vi "rsscope_core_global.vi"() -> ()   [LabVIEW 2014] (continued)
"Class Only"=FALSE, "Identifier"="RSSCOPE_ATTR_MASK_CONVERT_TO_USER", "Descriptive Name"="Mask Test Convert To User", "Data Type"=2, "Command"="MTES:CEM", "Access"=1, "Range Table"="", "Read Callback"="", "Write Callback"="", "Supported Models"="", "Instrument Options"="", "Flags"=0, "Help"="Converts the test and mask definitions of the current mask test to a new mask test of type User.\n\nAvailable Repeated Capabilities:\nNone\n\nRemote-control command(s):\nMTESt:CEMask"}, {"Level"=3, "Class Only"=FALSE, "Identifier"="RSSCOPE_ATTR_MASK_TEST_ENABLE", "Descriptive Name"="Mask Test Enable", "Data Type"=3, "Command"="MTES", "Access"=2, "Range Table"="", "Read Callback"="rsscope_formatMaskNameBoolean_ReadCallback.vi", "Write Callback"="rsscope_formatMaskNameBoolean_WriteCallback.vi", "Supported Models"="", "Instrument Options"="", "Flags"=0, "Help"="This attribute activates and deactivates the mask test.\n\nAvailable Repeated Capabilities:\nNone\n\nRemote-control command(s):\nMTESt[:STATe]"}, {"Level"=3, "Class Only"=FALSE, "Identifier"="RSSCOPE_ATTR_MASK_TEST_CLEAR_ALL", "Descriptive Name"="Mask Test Clear All", "Data Type"=4, "Command"="MTES:RST", "Access"=1, "Range Table"="", "Read Callback"="", "Write Callback"="", "Supported Models"="", "Instrument Options"="", "Flags"=0, "Help"="Clears all totals and results in all &apos;Mask Test&apos; result boxes.\n\nAvailable Repeated Capabilities:\nNone\n\nRemote-control command(s):\nMTESt:RST"}, {"Level"=3, "Class Only"=FALSE, "Identifier"="RSSCOPE_ATTR_MASK_TEST_DEFINITION_TYPE", "Descriptive Name"="Mask Test Definition Type", "Data Type"=0, "Command"="MTES:CTYP", "Access"=2, "Range Table"="RsScope_rngMaskTestDefinitionType", "Read Callback"="rsscope_formatMaskNameInt32_ReadCallback.vi", "Write Callback"="rsscope_formatMaskNameInt32_WriteCallback.vi", "Supported Models"="", "Instrument Options"="", "Flags"=0, "Help"="This control selects the method of mask definition.\n\nAvailable Repeated Capabilities:\nNone\n\nRemote-control command(s):\nMTESt:CTYPe"}, {"Level"=3, "Class Only"=FALSE, "Identifier"="RSSCOPE_ATTR_MASK_TEST_SOURCE", "Descriptive Name"="Mask Test Source", "Data Type"=0, "Command"="MTES:SOUR", "Access"=2, "Range Table"="rsscope_rngWaveformParameter", "Read Callback"="rsscope_formatMaskNameInt32_ReadCallback.vi", "Write Callback"="rsscope_formatMaskNameInt32_WriteCallback.vi", "Supported Models"="", "Instrument Options"="", "Flags"=0, "Help"="This attribute selects the waveform to be tested against the mask defined by RSSCOPE_ATTR_SELECTED_MASK_NAME.\n\nAvailable Repeated Capabilities:\nNone\n\nRemote-control command(s):\nMTESt:SOURce"}, {"Level"=3, "Class Only"=FALSE, "Identifier"="RSSCOPE_ATTR_MASK_TEST_FAIL_CONDITION", "Descriptive Name"="Mask Test Fail Condition", "Data Type"=0, "Command"="MTES:COND", "Access"=2, "Range Table"="RsScope_rngMaskTestFailCondition", "Read Callback"="rsscope_formatMaskNameInt32_ReadCallback.vi", "Write Callback"="rsscope_formatMaskNameInt32_WriteCallback.vi", "Supported Models"="", "Instrument Options"="", "Flags"=0, "Help"="Sets the first criteria for a failed test, the kind of hits to be considered for test evaluation.\n\nAvailable Repeated Capabilities:\nNone\n\nRemote-control command(s):\nMTESt:CONDition"}, {"Level"=3, "Class Only"=FALSE, "Identifier"="RSSCOPE_ATTR_MASK_TEST_VIOLATION_TOLERANCE", "Descriptive Name"="Mask Test Violation Tolerance", "Data Type"=5, "Command"="MTES:TOL", "Access"=2, "Range Table"="", "Read Callback"="rsscope_formatMaskNameInt64_ReadCallback.vi", "Write Callback"="rsscope_formatMaskNameInt64_WriteCallback.vi", "Supported Models"="", "Instrument Options"="", "Flags"=0, "Help"="Sets the second criteria for a failed test, the number of tolerable sample hits or acquisition hits.\n\nAvailable Repeated Capabilities:\nNone\n\nRemote-control command(s):\nMTESt:TOLerance"}, {"Level"=3, "Class Only"=FALSE, "Identifier"="RSSCOPE_ATTR_MASK_TEST_SAVE_PATH", "Descriptive Name"="Mask Test Save Path", "Data Type"=2, "Command"="MTES:FILE:NAME", "Access"=2, "Range Table"="", "Read Callback"="rsscope_formatMaskNameString_ReadCallback.vi", "Write Callback"="rsscope_formatMaskNameString_WriteCallback.vi", "Supported Models"="", "Instrument Options"="", "Flags"=0, "Help"="This attribute specifies a file to save the mask test.\n\nAvailable Repeated Capabilities:\nNone\n\nRemote-control command(s):\nMTESt:FILE:NAME"}, {"Level"=3, "Class Only"=FALSE, "Identifier"="RSSCOPE_ATTR_MASK_TEST_SAVE", "Descriptive Name"="Mask Test Save", "Data Type"=2, "Command"="MTES:FILE:SAVE", "Access"=1, "Range Table"="", "Read Callback"="", "Write Callback"="", "Supported Models"="", "Instrument Options"="", "Flags"=0, "Help"="Saves the mask test.\n\nAvailable Repeated Capabilities:\nNone\n\nRemote-control command(s):\nMTESt:FILE:SAVE"}, {"Level"=3, "Class Only"=FALSE, "Identifier"="RSSCOPE_ATTR_MASK_TEST_OPEN", "Descriptive Name"="Mask Test Open", "Data Type"=2, "Command"="MTES:FILE:OPEN", "Access"=1, "Range Table"="", "Read Callback"="", "Write Callback"="", "Supported Models"="", "Instrument Options"="", "Flags"=0, "Help"="Opens the mask test.\n\nAvailable Repeated Capabilities:\nNone\n\nRemote-control command(s):\nMTESt:FILE:OPEN"}, {"Level"=3, "Class Only"=FALSE, "Identifier"="RSSCOPE_ATTR_MASK_TEST_DELETE", "Descriptive Name"="Mask Test Delete", "Data Type"=2, "Command"="MTES:FILE:DEL", "Access"=1, "Range Table"="", "Read Callback"="", "Write Callback"="", "Supported Models"="", "Instrument Options"="", "Flags"=0, "Help"="Deletes the mask test.\n\nAvailable Repeated Capabilities:\nNone\n\nRemote-control command(s):\nMTESt:FILE:DELete"}, {"Level"=3, "Class Only"=FALSE, "Identifier"="RSSCOPE_ATTR_MASK_TEST_SEGMENT_CLEAR", "Descriptive Name"="Mask Test Segment Clear", "Data Type"=2, "Command"="MTES:SEGM:CLE", "Access"=1, "Range Table"="", "Read Callback"="", "Write Callback"="", "Supported Models"="", "Instrument Options"="", "Flags"=0, "Help"="Deletes all mask segments of the indicated mask test.\n\nAvailable Repeated Capabilities:\nNone\n\nRemote-control command(s):\nMTESt:SEGMent:CLEar"}, {"Level"=2, "Class Only"=TRUE, "Identifier"="", "Descriptive Name"="Mask Definition", "Data Type"=0, "Command"="", "Access"=0, "Range Table"="", "Read Callback"="", "Write Callback"="", "Supported Models"="", "Instrument Options"="", "Flags"=0, "Help"="Contains functionality for defining masks."}, {"Level"=3, "Class Only"=TRUE, "Identifier"="", "Descriptive Name"="User", "Data Type"=0, "Command"="", "Access"=0, "Range Table"="", "Read Callback"="", "Write Callback"="", "Supported Models"="", "Instrument Options"="", "Flags"=0, "Help"="A user mask is defined by entering the time and voltage values for all corner points of the\nmask segments. A user mask has at least one segment. Complex masks can have up to\n16 segments.\nAn inner segment is an area defined by three or more points. Upper and lower segments\nlimit the signal on top and bottom of the screen. They are defined by a line, the region\nabove or below the line is set automatically as mask segment."}, {"Level"=4, "Class Only"=FALSE, "Identifier"="RSSCOPE_ATTR_MASK_SELECTED_SEGMENT", "Descriptive Name"="Mask Selected Segment", "Data Type"=0, "Command"="", "Access"=2, "Range Table"="", "Read Callback"="", "Write Callback"="", "Supported Models"="", "Instrument Options"="", "Flags"=2, "Help"="Sets the segment that is in use.\n\nAvailable Repeated Capabilities:\nNone\n\nRemote-control command(s):\ncmd"}, {"Level"=4, "Class Only"=FALSE, "Identifier"="RSSCOPE_ATTR_MASK_SEGMENT_COUNT", "Descriptive Name"="Mask Segment Count", "Data Type"=0, "Command"="MTES:SEGM:COUN?", "Access"=0, "Range Table"="", "Read Callback"="rsscope_formatMaskNameInt32_ReadCallback.vi", "Write Callback"="", "Supported Models"="", "Instrument Options"="", "Flags"=0, "Help"="This attribute returns the number of segments in the mask definition.\n\nAvailable Repeated Capabilities:\nNone\n\nRemote-control command(s):\nMTESt:SEGMent:COUNt?"}, {"Level"=4, "Class Only"=TRUE, "Identifier"="", "Descriptive Name"="Segment", "Data Type"=0, "Command"="", "Access"=0, "Range Table"="", "Read Callback"="", "Write Callback"="", "Supported Models"="", "Instrument Options"="", "Flags"=0, "Help"="This clas contains attributes, in which segments are selected using SelectedSegment."}, {"Level"=5, "Class Only"=FALSE, "Identifier"="RSSCOPE_ATTR_MASK_SEGMENT_ADD", "Descriptive Name"="Mask Segment Add", "Data Type"=2, "Command"="MTES:SEGM:ADD", "Access"=1, "Range Table"="", "Read Callback"="", "Write Callback"="", "Supported Models"="", "Instrument Options"="", "Flags"=0, "Help"="Creates a new segment in the mask definition.\n\nAvailable Repeated Capabilities:\nNone\n\nRemote-control command(s):\nMTESt:SEGMent:ADD"}, {"Level"=5, "Class Only"=FALSE, "Identifier"="RSSCOPE_ATTR_MASK_SELECTED_POINT", "Descriptive Name"="Mask Selected Point", "Data Type"=0, "Command"="", "Access"=2, "Range Table"="", "Read Callback"="", "Write Callback"="", "Supported Models"="", "Instrument Options"="", "Flags"=2, "Help"="Sets the point that is in use.\n\nAvailable Repeated Capabilities:\nNone\n\nRemote-control command(s):\ncmd"}, {"Level"=5, "Class Only"=TRUE, "Identifier"="", "Descriptive Name"="Point", "Data Type"=0, "Command"="", "Access"=0, "Range Table"="", "Read Callback"="", "Write Callback"="", "Supported Models"="", "Instrument Options"="", "Flags"=0, "Help"="This clas contains attributes, in which points are selected using SelectedPoint."}, {"Level"=3, "Class Only"=TRUE, "Identifier"="", "Descriptive Name"="Waveform", "Data Type"=0, "Command"="", "Access"=0, "Range Table"="", "Read Callback"="", "Write Callback"="", "Supported Models"="", "Instrument Options"="", "Flags"=0, "Help"="A waveform mask is created from an existing waveform. The waveform builds the upper\nand lower limit line of the mask, and the limits are moved and stretched. The result is a\ntolerance tube around the waveform that is used as mask."}, {"Level"=4, "Class Only"=FALSE, "Identifier"="RSSCOPE_ATTR_MASK_COPY_WAVEFORM", "Descriptive Name"="Mask Copy Waveform", "Data Type"=2, "Command"="MTES:WFMLupdate", "Access"=1, "Range Table"="", "Read Callback"="", "Write Callback"="", "Supported Models"="", "Instrument Options"="", "Flags"=0, "Help"="Creates the upper and lower mask limit from the envelope of the selected reference waveform.\n\nAvailable Repeated Capabilities:\nNone\n\nRemote-control command(s):\nMTESt:WFMLupdate"}, {"Level"=4, "Class Only"=FALSE, "Identifier"="RSSCOPE_ATTR_MASK_WAVEFORM_USED_REFERENCE", "Descriptive Name"="Mask Waveform Used Reference", "Data Type"=0, "Command"="MTES:REFW", "Access"=2, "Range Table"="RsScope_rngMaskWaveformUsedReference", "Read Callback"="rsscope_formatMaskNameInt32_ReadCallback.vi", "Write Callback"="rsscope_formatMaskNameInt32_WriteCallback.vi", "Supported Models"="", "Instrument Options"="", "Flags"=0, "Help"="Sets the reference waveform from which the mask is created.\n\nAvailable Repeated Capabilities:\nNone\n\nRemote-control command(s):\nMTESt:REFWfm"}, {"Level"=4, "Class Only"=FALSE, "Identifier"="RSSCOPE_ATTR_MASK_WAVEFORM_HORIZONTAL_WIDTH", "Descriptive Name"="Mask Waveform Horizontal Width", "Data Type"=1, "Command"="MTES:WFMR:XWID", "Access"=2, "Range Table"="RsScope_rngMaskWaveformWidth", "Read Callback"="rsscope_formatMaskNameReal64_ReadCallback.vi", "Write Callback"="rsscope_formatMaskNameReal64_WriteCallback.vi", "Supported Models"="", "Instrument Options"="", "Flags"=0, "Help"="Sets the width of the mask in horizontal direction. The specified number of divisions is added to the positive x-values and subtracted from the negative x-values of the mask limits in relation to the source waveform of the mask. The overall mask width is twice the specified horizontal width.\n\nAvailable Repeated Capabilities:\nNone\n\nRemote-control command(s):\nMTESt:WFMRescale:XWIDth"}, {"Level"=4, "Class Only"=FALSE, "Identifier"="RSSCOPE_ATTR_MASK_WAVEFORM_VERTICAL_WIDTH", "Descriptive Name"="Mask Waveform Vertical Width", "Data Type"=1, "Command"="MTES:WFMR:YWID", "Access"=2, "Range Table"="RsScope_rngMaskWaveformWidth", "Read Callback"="rsscope_formatMaskNameReal64_ReadCallback.vi", "Write Callback"="rsscope_formatMaskNameReal64_WriteCallback.vi", "Supported Models"="", "Instrument Options"="", "Flags"=0, "Help"="Sets the width of the waveform mask in vertical direction. The specified number of divisions is added to the y-values of the upper mask limit and subtracted from the y-values of the lower mask limit. Thus, the upper half of the mask is pulled upwards, the lower half is pulled down, and the overall height of the mask is twice the vertical width.\n\nAvailable Repeated Capabilities:\nNone\n\nRemote-control command(s):\nMTESt:WFMRescale:YWIDth"}, {"Level"=4, "Class Only"=FALSE, "Identifier"="RSSCOPE_ATTR_MASK_WAVEFORM_VERTICAL_STRETCH", "Descriptive Name"="Mask Waveform Vertical Stretch", "Data Type"=0, "Command"="MTES:WFMR:YSTR", "Access"=2, "Range Table"="RsScope_rngMaskWaveformVerticalStretch", "Read Callback"="rsscope_formatMaskNameInt32_ReadCallback.vi", "Write Callback"="rsscope_formatMaskNameInt32_WriteCallback.vi", "Supported Models"="", "Instrument Options"="", "Flags"=0, "Help"="This control sets the vertical scaling to stretch the mask in y-direction. The scaling axis is the horizontal line through the lowest value of the lower mask limit.\n\nAvailable Repeated Capabilities:\nNone\n\nRemote-control command(s):\nMTESt:WFMRescale:YSTRetch"}, {"Level"=4, "Class Only"=FALSE, "Identifier"="RSSCOPE_ATTR_MASK_WAVEFORM_VERTICAL_POSITION", "Descriptive Name"="Mask Waveform Vertical Position", "Data Type"=1, "Command"="MTES:WFMR:YPOS", "Access"=2, "Range Table"="RsScope_rngMaskWaveformVerticalPosition", "Read Callback"="rsscope_formatMaskNameReal64_ReadCallback.vi", "Write Callback"="rsscope_formatMaskNameReal64_WriteCallback.vi", "Supported Models"="", "Instrument Options"="", "Flags"=0, "Help"="This attribute moves the mask vertically within the display.\n\nAvailable Repeated Capabilities:\nNone\n\nRemote-control command(s):\nMTESt:WFMRescale:YPOSition"}, {"Level"=3, "Class Only"=TRUE, "Identifier"="", "Descriptive Name"="Eye", "Data Type"=0, "Command"="", "Access"=0, "Range Table"="", "Read Callback"="", "Write Callback"="", "Supported Models"="", "Instrument Options"="", "Flags"=0, "Help"="Mask testing on eye diagrams allows you to test data signals against eye shapes that are\nrequired in the standards. You can select the shape of the eye, enter its dimensions and\nposition the eye on the display."}, {"Level"=4, "Class Only"=FALSE, "Identifier"="RSSCOPE_ATTR_MASK_TEST_EYE_SHAPE", "Descriptive Name"="Mask Test Eye Shape", "Data Type"=0, "Command"="MTES:EYEM:TYPE", "Access"=2, "Range Table"="RsScope_rngMaskTestEyeShape", "Read Callback"="rsscope_formatMaskNameInt32_ReadCallback.vi", "Write Callback"="rsscope_formatMaskNameInt32_WriteCallback.vi", "Supported Models"="", "Instrument Options"="K12", "Flags"=0, "Help"="This attribute defines the outline of the eye mask.\n\nAvailable Repeated Capabilities:\nNone\n\nRemote-control command(s):\nMTESt:EYEMask:TYPE"}, {"Level"=4, "Class Only"=FALSE, "Identifier"="RSSCOPE_ATTR_MASK_TEST_EYE_MAIN_WIDTH", "Descriptive Name"="Mask Test Eye Main Width", "Data Type"=1, "Command"="MTES:EYEM:WIDTh1", "Access"=2, "Range Table"="", "Read Callback"="rsscope_formatMaskNameReal64_ReadCallback.vi", "Write Callback"="rsscope_formatMaskNameReal64_WriteCallback.vi", "Supported Models"="", "Instrument Options"="K12", "Flags"=0, "Help"="Main width defines the width af all eye mask shapes.\n\nAvailable Repeated Capabilities:\nNone\n\nRemote-control command(s):\nMTESt:EYEMask:WIDTh<m>[:VALue]"}, {"Level"=4, "Class Only"=FALSE, "Identifier"="RSSCOPE_ATTR_MASK_TEST_EYE_MINOR_WIDTH", "Descriptive Name"="Mask Test Eye Minor Width", "Data Type"=1, "Command"="MTES:EYEM:WIDTh2", "Access"=2, "Range Table"="", "Read Callback"="rsscope_formatMaskNameReal64_ReadCallback.vi", "Write Callback"="rsscope_formatMaskNameReal64_WriteCallback.vi", "Supported Models"="", "Instrument Options"="K12", "Flags"=0, "Help"="Minor width defines the secondary width for hexagon and octagon mask shapes.\n\nAvailable Repeated Capabilities:\nNone\n\nRemote-control command(s):\nMTESt:EYEMask:WIDTh<m>[:VALue]"}, {"Level"=4, "Class Only"=FALSE, "Identifier"="RSSCOPE_ATTR_MASK_TEST_EYE_MAIN_HEIGHT", "Descriptive Name"="Mask Test Eye Main Height", "Data Type"=1, "Command"="MTES:EYEM:HEIGht1", "Access"=2, "Range Table"="", "Read Callback"="rsscope_formatMaskNameReal64_ReadCallback.vi", "Write Callback"="rsscope_formatMaskNameReal64_WriteCallback.vi", "Supported Models"="", "Instrument Options"="K12", "Flags"=0, "Help"="Main height defines the heigth af all eye mask shapes.\n\nAvailable Repeated Capabilities:\nNone\n\nRemote-control command(s):\nMTESt:EYEMask:HEIGht<m>[:VALue]"}, {"Level"=4, "Class Only"=FALSE, "Identifier"="RSSCOPE_ATTR_MASK_TEST_EYE_MINOR_HEIGHT", "Descriptive Name"="Mask Test Eye Minor Height", "Data Type"=1, "Command"="MTES:EYEM:HEIGht2", "Access"=2, "Range Table"="", "Read Callback"="rsscope_formatMaskNameReal64_ReadCallback.vi", "Write Callback"="rsscope_formatMaskNameReal64_WriteCallback.vi", "Supported Models"="", "Instrument Options"="K12", "Flags"=0, "Help"="Minor height defines the secondary height for octagon mask shapes.\n\nAvailable Repeated Capabilities:\nNone\n\nRemote-control command(s):\nMTESt:EYEMask:HEIGht<m>[:VALue]"}, {"Level"=4, "Class Only"=FALSE, "Identifier"="RSSCOPE_ATTR_MASK_TEST_EYE_COPY_LEFT", "Descriptive Name"="Mask Test Eye Copy Left", "Data Type"=3, "Command"="MTES:EYEM:MSKL", "Access"=2, "Range Table"="", "Read Callback"="rsscope_formatMaskNameBoolean_ReadCallback.vi", "Write Callback"="rsscope_formatMaskNameBoolean_WriteCallback.vi", "Supported Models"="", "Instrument Options"="K12", "Flags"=0, "Help"="Copies the eye shape to the left.\n\nAvailable Repeated Capabilities:\nNone\n\nRemote-control command(s):\nMTESt:EYEMask:MSKLeft"}, {"Level"=4, "Class Only"=FALSE, "Identifier"="RSSCOPE_ATTR_MASK_TEST_EYE_COPY_RIGHT", "Descriptive Name"="Mask Test Eye Copy Right", "Data Type"=3, "Command"="MTES:EYEM:MSKR", "Access"=2, "Range Table"="", "Read Callback"="rsscope_formatMaskNameBoolean_ReadCallback.vi", "Write Callback"="rsscope_formatMaskNameBoolean_WriteCallback.vi", "Supported Models"="", "Instrument Options"="K12", "Flags"=0, "Help"="Copies the eye shape to the right.\n\nAvailable Repeated Capabilities:\nNone\n\nRemote-control command(s):\nMTESt:EYEMask:MSKRight"}, {"Level"=4, "Class Only"=FALSE, "Identifier"="RSSCOPE_ATTR_MASK_TEST_EYE_INTERPATTERN_LENGTH", "Descriptive Name"="Mask Test Eye Interpattern Length", "Data Type"=1, "Command"="MTES:EYEM:HPER", "Access"=2, "Range Table"="RsScope_rngMaskTestEyeInterpatternLength", "Read Callback"="rsscope_formatMaskNameReal64_ReadCallback.vi", "Write Callback"="rsscope_formatMaskNameReal64_WriteCallback.vi", "Supported Models"="", "Instrument Options"="K12", "Flags"=0, "Help"="Defines the time distance between the shape centers if Copy Left and/or Copy Right are On.\n\nAvailable Repeated Capabilities:\nNone\n\nRemote-control command(s):\nMTESt:EYEMask:HPERiod"}, {"Level"=4, "Class Only"=FALSE, "Identifier"="RSSCOPE_ATTR_MASK_TEST_EYE_TOP_ENABLE", "Descriptive Name"="Mask Test Eye Top Enable", "Data Type"=3, "Command"="MTES:EYEM:MSKT", "Access"=2, "Range Table"="", "Read Callback"="rsscope_formatMaskNameBoolean_ReadCallback.vi", "Write Callback"="rsscope_formatMaskNameBoolean_WriteCallback.vi", "Supported Models"="", "Instrument Options"="K12", "Flags"=0, "Help"="Enable the lower (bottom) mask region.\n\nAvailable Repeated Capabilities:\nNone\n\nRemote-control command(s):\nMTESt:EYEMask:MSKTop"}, {"Level"=4, "Class Only"=FALSE, "Identifier"="RSSCOPE_ATTR_MASK_TEST_EYE_BOTTOM_ENABLE", "Descriptive Name"="Mask Test Eye Bottom Enable", "Data Type"=3, "Command"="MTES:EYEM:MSKB", "Access"=2, "Range Table"="", "Read Callback"="rsscope_formatMaskNameBoolean_ReadCallback.vi", "Write Callback"="rsscope_formatMaskNameBoolean_WriteCallback.vi", "Supported Models"="", "Instrument Options"="K12", "Flags"=0, "Help"="Enable the lower (bottom) mask region.\n\nAvailable Repeated Capabilities:\nNone\n\nRemote-control command(s):\nMTESt:EYEMask:MSKBottom"}, {"Level"=4, "Class Only"=FALSE, "Identifier"="RSSCOPE_ATTR_MASK_TEST_EYE_OFFSET_TOP", "Descriptive Name"="Mask Test Eye Offset Top", "Data Type"=1, "Command"="MTES:EYEM:TOFF", "Access"=2, "Range Table"="RsScope_rngMaskEyeOffset", "Read Callback"="rsscope_formatMaskNameReal64_ReadCallback.vi", "Write Callback"="rsscope_formatMaskNameReal64_WriteCallback.vi", "Supported Models"="", "Instrument Options"="K12", "Flags"=0, "Help"="Defines the time distance between the shape centers if Copy Left and/or Copy Right are On.\n\nAvailable Repeated Capabilities:\nNone\n\nRemote-control command(s):\nMTESt:EYEMask:TOFFset"}, {"Level"=4, "Class Only"=FALSE, "Identifier"="RSSCOPE_ATTR_MASK_TEST_EYE_OFFSET_BOTTOM", "Descriptive Name"="Mask Test Eye Offset Bottom", "Data Type"=1, "Command"="MTES:EYEM:BOFF", "Access"=2, "Range Table"="RsScope_rngMaskEyeOffset", "Read Callback"="rsscope_formatMaskNameReal64_ReadCallback.vi", "Write Callback"="rsscope_formatMaskNameReal64_WriteCallback.vi", "Supported Models"="", "Instrument Options"="K12", "Flags"=0, "Help"="Voltage distance from the eye shape center that limit the lower regions.\n\nAvailable Repeated Capabilities:\nNone\n\nRemote-control command(s):\nMTESt:EYEMask:BOFFset"}, {"Level"=4, "Class Only"=FALSE, "Identifier"="RSSCOPE_ATTR_MASK_TEST_EYE_TIME_WIDTH", "Descriptive Name"="Mask Test Eye Time Width", "Data Type"=1, "Command"="MTES:EYEM:TBW", "Access"=2, "Range Table"="RsScope_rngMaskEyeTimeWidth", "Read Callback"="rsscope_formatMaskNameReal64_ReadCallback.vi", "Write Callback"="rsscope_formatMaskNameReal64_WriteCallback.vi", "Supported Models"="", "Instrument Options"="K12", "Flags"=0, "Help"="Time width of the outer regions, symmetric to the eye shape center.\n\nAvailable Repeated Capabilities:\nNone\n\nRemote-control command(s):\nMTESt:EYEMask:TBWidth"}, {"Level"=4, "Class Only"=FALSE, "Identifier"="RSSCOPE_ATTR_MASK_TEST_EYE_SYMETRIC", "Descriptive Name"="Mask Test Eye Symetric", "Data Type"=3, "Command"="MTES:EYEM:TBSY", "Access"=2, "Range Table"="", "Read Callback"="rsscope_formatMaskNameBoolean_ReadCallback.vi", "Write Callback"="rsscope_formatMaskNameBoolean_WriteCallback.vi", "Supported Models"="", "Instrument Options"="K12", "Flags"=0, "Help"="Sets bottom and top offsets to the same value so that the outer regions are symmetric to the eye shape.\n\nAvailable Repeated Capabilities:\nNone\n\nRemote-control command(s):\nMTESt:EYEMask:TBSYmmetric"}, {"Level"=4, "Class Only"=FALSE, "Identifier"="RSSCOPE_ATTR_MASK_TEST_EYE_HORIZONTAL_POSITION", "Descriptive Name"="Mask Test Eye Horizontal Position", "Data Type"=1, "Command"="MTES:EYEM:HPOS", "Access"=2, "Range Table"="RsScope_rngMaskEyePosition", "Read Callback"="rsscope_formatMaskNameReal64_ReadCallback.vi", "Write Callback"="rsscope_formatMaskNameReal64_WriteCallback.vi", "Supported Models"="", "Instrument Options"="K12", "Flags"=0, "Help"="Sets the horizontal (time) value of the eye shape enter and thus defines the horizontal position of the eye shape on the display.\n\nAvailable Repeated Capabilities:\nNone\n\nRemote-control command(s):\nMTESt:EYEMask:HPOSition"}, {"Level"=4, "Class Only"=FALSE, "Identifier"="RSSCOPE_ATTR_MASK_TEST_EYE_VERTICAL_POSITION", "Descriptive Name"="Mask Test Eye Vertical Position", "Data Type"=1, "Command"="MTES:EYEM:VPOS", "Access"=2, "Range Table"="RsScope_rngMaskEyePosition", "Read Callback"="rsscope_formatMaskNameReal64_ReadCallback.vi", "Write Callback"="rsscope_formatMaskNameReal64_WriteCallback.vi", "Supported Models"="", "Instrument Options"="K12", "Flags"=0, "Help"="Sets the vertical (voltage) value of the eye shape enter and thus defines the vertical position of the eye shape on the display.\n\nAvailable Repeated Capabilities:\nNone\n\nRemote-control command(s):\nMTESt:EYEMask:VPOSition"}, {"Level"=2, "Class Only"=TRUE, "Identifier"="", "Descriptive Name"="Mask Display", "Data Type"=0, "Command"="", "Access"=0, "Range Table"="", "Read Callback"="", "Write Callback"="", "Supported Models"="", "Instrument Options"="", "Flags"=0, "Help"="Contains settings for mask and hit display."}, {"Level"=3, "Class Only"=FALSE, "Identifier"="RSSCOPE_ATTR_MASK_TEST_LABEL_STATE", "Descriptive Name"="Mask Test Label State", "Data Type"=3, "Command"="MTES:LAB", "Access"=2, "Range Table"="", "Read Callback"="", "Write Callback"="", "Supported Models"="", "Instrument Options"="", "Flags"=0, "Help"="Switches the display of the mask test name on or off.\n\nAvailable Repeated Capabilities:\nNone\n\nRemote-control command(s):\nMTESt:LABel"}, {"Level"=3, "Class Only"=FALSE, "Identifier"="RSSCOPE_ATTR_MASK_TEST_RENAME", "Descriptive Name"="Mask Test Rename", "Data Type"=2, "Command"="MTES:REN", "Access"=2, "Range Table"="", "Read Callback"="rsscope_formatMaskNameString_ReadCallback.vi", "Write Callback"="rsscope_formatMaskNameString_WriteCallback.vi", "Supported Models"="", "Instrument Options"="", "Flags"=0, "Help"="Changes the name of the mask test.\n\nAvailable Repeated Capabilities:\nNone\n\nRemote-control command(s):\nMTESt:REName"}, {"Level"=3, "Class Only"=FALSE, "Identifier"="RSSCOPE_ATTR_MASK_TEST_HIGHLIGHT_STATE", "Descriptive Name"="Mask Test Highlight State", "Data Type"=3, "Command"="MTES:HIGH:STAT", "Access"=2, "Range Table"="", "Read Callback"="", "Write Callback"="", "Supported Models"="", "Instrument Options"="", "Flags"=0, "Help"="If ON, the mask hits are highlighted on the screen. You can define the color and the time of the hit display.\n\nAvailable Repeated Capabilities:\nNone\n\nRemote-control command(s):\nMTESt:HIGHlight:STATe"}, {"Level"=3, "Class Only"=FALSE, "Identifier"="RSSCOPE_ATTR_MASK_TEST_HIGHLIGHT_TIME", "Descriptive Name"="Mask Test Highlight Time", "Data Type"=1, "Command"="MTES:HIGH:TIME", "Access"=2, "Range Table"="RsScope_rngMaskTestHighlightTime", "Read Callback"="", "Write Callback"="", "Supported Models"="", "Instrument Options"="", "Flags"=0, "Help"="Sets the time how long the mask hits are highlighted.\n\nAvailable Repeated Capabilities:\nNone\n\nRemote-control command(s):\nMTESt:HIGHlight:TIME"}, {"Level"=3, "Class Only"=FALSE, "Identifier"="RSSCOPE_ATTR_MASK_TEST_HIGHLIGHT_ENDLESS", "Descriptive Name"="Mask Test Highlight Endless", "Data Type"=3, "Command"="MTES:HIGH:INF", "Access"=2, "Range Table"="", "Read Callback"="", "Write Callback"="", "Supported Models"="", "Instrument Options"="", "Flags"=0, "Help"="If TRUE, the mask hits are highlighted for an unlimited period of time.\n\nAvailable Repeated Capabilities:\nNone\n\nRemote-control command(s):\nMTESt:HIGHlight:INFinite"}, {"Level"=3, "Class Only"=FALSE, "Identifier"="RSSCOPE_ATTR_MASK_TEST_COLOR_UNMATCHED", "Descriptive Name"="Mask Test Color Unmatched", "Data Type"=5, "Command"="MTES:COL:UNM", "Access"=2, "Range Table"="RsScope_rngARGB", "Read Callback"="", "Write Callback"="", "Supported Models"="", "Instrument Options"="", "Flags"=0, "Help"="Sets the color of masks segments that were not hit.\n\nAvailable Repeated Capabilities:\nNone\n\nRemote-control command(s):\nMTESt:COLor:UNMatch"}, {"Level"=3, "Class Only"=FALSE, "Identifier"="RSSCOPE_ATTR_MASK_TEST_COLOR_MATCHED", "Descriptive Name"="Mask Test Color Matched", "Data Type"=5, "Command"="MTES:COL:MATC", "Access"=2, "Range Table"="RsScope_rngARGB", "Read Callback"="", "Write Callback"="", "Supported Models"="", "Instrument Options"="", "Flags"=0, "Help"="Sets the color of samples that violated the mask.\n\nAvailable Repeated Capabilities:\nNone\n\nRemote-control command(s):\nMTESt:COLor:MATCh"}, {"Level"=3, "Class Only"=FALSE, "Identifier"="RSSCOPE_ATTR_MASK_TEST_COLOR_BORDER", "Descriptive Name"="Mask Test Color Border", "Data Type"=5, "Command"="MTES:COL:BORD", "Access"=2, "Range Table"="RsScope_rngARGB", "Read Callback"="", "Write Callback"="", "Supported Models"="", "Instrument Options"="", "Flags"=0, "Help"="Sets the color of masks segments that were touched at the border. In this case, the resolution is not sufficient to detect if the mask was really hit or not. Zoom into the concerned area to see the actual result.\n\nAvailable Repeated Capabilities:\nNone\n\nRemote-control command(s):\nMTESt:COLor:BORDer"}, {"Level"=3, "Class Only"=FALSE, "Identifier"="RSSCOPE_ATTR_MASK_TEST_COLOR_INTERIOR", "Descriptive Name"="Mask Test Color Interior", "Data Type"=5, "Command"="MTES:COL:INT", "Access"=2, "Range Table"="RsScope_rngARGB", "Read Callback"="", "Write Callback"="", "Supported Models"="", "Instrument Options"="", "Flags"=0, "Help"="Sets the color of mask segments the signal has entered into.\n\nAvailable Repeated Capabilities:\nNone\n\nRemote-control command(s):\nMTESt:COLor:INTerior"}, {"Level"=1, "Class Only"=TRUE, "Identifier"="", "Descriptive Name"="Search", "Data Type"=0, "Command"="", "Access"=0, "Range Table"="", "Read Callback"="", "Write Callback"="", "Supported Models"="", "Instrument Options"="", "Flags"=0, "Help"="Search functions allow you to detect and analyze specific conditions in the acquired data\nquickly and simply. This is possible both for running acquisitions or for waveforms stored\nin the sample memory, or for an extract of either. Various search conditions are available,\nincluding trigger parameters such as edges, windows or states. Search results can then\nbe qualified further by other waveform conditions."}, {"Level"=2, "Class Only"=FALSE, "Identifier"="RSSCOPE_ATTR_SELECTED_SEARCH_NAME", "Descriptive Name"="Selected Search Name", "Data Type"=2, "Command"="", "Access"=2, "Range Table"="", "Read Callback"="", "Write Callback"="", "Supported Models"="", "Instrument Options"="", "Flags"=2, "Help"="This attribute selects the search name used for following attributes.\n\nAvailable Repeated Capabilities:\nNone\n\nRemote-control command(s):\n"}, {"Level"=2, "Class Only"=FALSE, "Identifier"="RSSCOPE_ATTR_SELECTED_SEARCH_SOURCE", "Descriptive Name"="Selected Search Source", "Data Type"=0, "Command"="", "Access"=2, "Range Table"="RsScope_rngSearchSource", "Read Callback"="", "Write Callback"="", "Supported Models"="", "Instrument Options"="", "Flags"=2, "Help"="Sets Search Source selector.\n\nAvailable Repeated Capabilities:\nNone\n\nRemote-control command(s):\ncmd"}, {"Level"=2, "Class Only"=FALSE, "Identifier"="RSSCOPE_ATTR_NEW_SEARCH", "Descriptive Name"="New Search", "Data Type"=2, "Command"="SEAR:ADD", "Access"=1, "Range Table"="", "Read Callback"="", "Write Callback"="", "Supported Models"="", "Instrument Options"="", "Flags"=0, "Help"="Creates a new search definition with the specified name.\n\nAvailable Repeated Capabilities:\nNone\n\nRemote-control command(s):\nSEARch:ADD"}, {"Level"=2, "Class Only"=FALSE, "Identifier"="RSSCOPE_ATTR_DELETE_SEARCH", "Descriptive Name"="Delete Search", "Data Type"=2, "Command"="SEAR:REM", "Access"=1, "Range Table"="", "Read Callback"="", "Write Callback"="", "Supported Models"="", "Instrument Options"="", "Flags"=0, "Help"="Deletes the specified search definition.\n\nAvailable Repeated Capabilities:\nNone\n\nRemote-control command(s):\nSEARch:REMove"}, {"Level"=2, "Class Only"=FALSE, "Identifier"="RSSCOPE_ATTR_SEARCH_NEXT_RESULT", "Descriptive Name"="Search Next Result", "Data Type"=2, "Command"="SEAR:NEXT", "Access"=1, "Range Table"="", "Read Callback"="", "Write Callback"="", "Supported Models"="", "Instrument Options"="", "Flags"=0, "Help"="Performs a single search for the next result on the existing data from the selected source.\n\nAvailable Repeated Capabilities:\nNone\n\nRemote-control command(s):\nSEARch:NEXT"}, {"Level"=2, "Class Only"=FALSE, "Identifier"="RSSCOPE_ATTR_SEARCH_ALL_RESULTS", "Descriptive Name"="Search All Results", "Data Type"=2, "Command"="SEAR:ALL", "Access"=1, "Range Table"="", "Read Callback"="", "Write Callback"="", "Supported Models"="", "Instrument Options"="", "Flags"=0, "Help"="Performs a search for all results on the existing data from the selected source.\n\nAvailable Repeated Capabilities:\nNone\n\nRemote-control command(s):\nSEARch:ALL"}, {"Level"=2, "Class Only"=FALSE, "Identifier"="RSSCOPE_ATTR_CLEAR_SEARCH_RESULTS", "Descriptive Name"="Clear Search Results", "Data Type"=2, "Command"="SEAR:CLE", "Access"=1, "Range Table"="", "Read Callback"="", "Write Callback"="", "Supported Models"="", "Instrument Options"="", "Flags"=0, "Help"="Clears the search results once to start a new search.\n\nAvailable Repeated Capabilities:\nNone\n\nRemote-control command(s):\nSEARch:CLEar"}, {"Level"=2, "Class Only"=FALSE, "Identifier"="RSSCOPE_ATTR_SEARCH_TRIGGER_LEVEL_AUTO_FIND", "Descriptive Name"="Search Trigger Level Auto Find", "Data Type"=2, "Command"="SEAR:TRIG:FIND", "Access"=1, "Range Table"="", "Read Callback"="", "Write Callback"="", "Supported Models"="", "Instrument Options"="", "Flags"=0, "Help"="Sets the trigger level automatically to 0.5 * (MaxPeak  MinPeak). The attribute is not available for an external trigger source.\n\nAvailable Repeated Capabilities:\nNone\n\nRemote-control command(s):\nSEARch:TRIGger:FINDlevel"}, {"Level"=2, "Class Only"=FALSE, "Identifier"="RSSCOPE_ATTR_SEARCH_SOURCE", "Descriptive Name"="Search Source", "Data Type"=0, "Command"="SEAR:SOUR", "Access"=2, "Range Table"="RsScope_rngSearchSource", "Read Callback"="rsscope_FormatSearchNameInt32_ReadCallback.vi", "Write Callback"="rsscope_FormatSearchNameInt32_WriteCallback.vi", "Supported Models"="", "Instrument Options"="", "Flags"=0, "Help"="Defines the source on which the search conditions are applied. The source can be any analog or digital channel, math or reference waveform.\n\nAvailable Repeated Capabilities:\nNone\n\nRemote-control command(s):\nSEARch:SOURce"}, {"Level"=2, "Class Only"=FALSE, "Identifier"="RSSCOPE_ATTR_SEARCH_ONLINE", "Descriptive Name"="Search Online", "Data Type"=3, "Command"="SEAR:ONL", "Access"=2, "Range Table"="", "Read Callback"="rsscope_FormatSearchNameBoolean_ReadCallback.vi", "Write Callback"="rsscope_FormatSearchNameBoolean_WriteCallback.vi", "Supported Models"="", "Instrument Options"="", "Flags"=0, "Help"="If enabled, a search is performed repeatedly for each new data acquisition.\n\nAvailable Repeated Capabilities:\nNone\n\nRemote-control command(s):\nSEARch:ONLine"}, {"Level"=2, "Class Only"=TRUE, "Identifier"="", "Descriptive Name"="Trigger", "Data Type"=0, "Command"="", "Access"=0, "Range Table"="", "Read Callback"="", "Write Callback"="", "Supported Models"="", "Instrument Options"="", "Flags"=0, "Help"="For trigger searches, most parameters available for trigger event definition can also be\nconfigured as search conditions. However, not only signal channels, but also math and\nreference waveforms can be selected as the search source. Each event type is defined\nin a separate tab. You can enable several event types for simultaneous search."}, {"Level"=3, "Class Only"=FALSE, "Identifier"="RSSCOPE_ATTR_SEARCH_TRIGGER_LEVEL", "Descriptive Name"="Search Trigger Level", "Data Type"=1, "Command"="SEAR:TRIG:LEV", "Access"=2, "Range Table"="", "Read Callback"="rsscope_FormatSearchNameSourceReal64_ReadCallback.vi", "Write Callback"="rsscope_FormatSearchNameSourceReal64_WriteCallback.vi", "Supported Models"="", "Instrument Options"="", "Flags"=0, "Help"="Sets the voltage level for the trigger level that is used to determine other parameters. Set the applicable search name with RSSCOPE_ATTR_SELECTED_SEARCH_NAME and the applicable search source with RSSCOPE_ATTR_SELECTED_SEARCH_SOURCE before using this attribute.\n\nAvailable Repeated Capabilities:\nNone\n\nRemote-control command(s):\nSEARch:TRIGger:LEVel[:VALue]"}, {"Level"=3, "Class Only"=FALSE, "Identifier"="RSSCOPE_ATTR_SEARCH_TRIGGER_CONDITIONS", "Descriptive Name"="Search Trigger Conditions", "Data Type"=2, "Command"="SEAR:TRIG:COND?", "Access"=0, "Range Table"="", "Read Callback"="rsscope_FormatSearchNameString_ReadCallback.vi", "Write Callback"="rsscope_FormatSearchNameString_WriteCallback.vi", "Supported Models"="", "Instrument Options"="", "Flags"=0, "Help"="This attribute returns the trigger search condition. It provides logical combinations of the input channels, math or reference waveforms, and supports you in verifying the operation of digital logic.\n\nAvailable Repeated Capabilities:\nNone\n\nRemote-control command(s):\nSEARch:TRIGger:CONDitions?"}, {"Level"=3, "Class Only"=TRUE, "Identifier"="", "Descriptive Name"="Edge", "Data Type"=0, "Command"="", "Access"=0, "Range Table"="", "Read Callback"="", "Write Callback"="", "Supported Models"="", "Instrument Options"="", "Flags"=0, "Help"="Configures the conditions for the edge trigger search.  An edge trigger occurs when the trigger signal passes through the voltage threshold that you specify with the Trigger Level parameter and has the slope that you specify with the Trigger Slope parameter."}, {"Level"=4, "Class Only"=FALSE, "Identifier"="RSSCOPE_ATTR_SEARCH_TRIGGER_EDGE_ENABLED", "Descriptive Name"="Search Trigger Edge Enabled", "Data Type"=3, "Command"="SEAR:TRIG:EDGE", "Access"=2, "Range Table"="", "Read Callback"="rsscope_FormatSearchNameBoolean_ReadCallback.vi", "Write Callback"="rsscope_FormatSearchNameBoolean_WriteCallback.vi", "Supported Models"="", "Instrument Options"="", "Flags"=0, "Help"="Includes the search conditions for the edge trigger event type in the next search.\n\nAvailable Repeated Capabilities:\nNone\n\nRemote-control command(s):\nSEARch:TRIGger:EDGE[:STATe]"}, {"Level"=4, "Class Only"=FALSE, "Identifier"="RSSCOPE_ATTR_SEARCH_TRIGGER_EDGE_SLOPE", "Descriptive Name"="Search Trigger Edge Slope", "Data Type"=0, "Command"="SEAR:TRIG:EDGE:SLOP", "Access"=2, "Range Table"="rsscope_rngTriggerSlope", "Read Callback"="rsscope_FormatSearchNameInt32_ReadCallback.vi", "Write Callback"="rsscope_FormatSearchNameInt32_WriteCallback.vi", "Supported Models"="", "Instrument Options"="", "Flags"=0, "Help"="Selects the edge type.\n\nAvailable Repeated Capabilities:\nNone\n\nRemote-control command(s):\nSEARch:TRIGger:EDGE:SLOPe"}, {"Level"=4, "Class Only"=FALSE, "Identifier"="RSSCOPE_ATTR_SEARCH_TRIGGER_EDGE_COPY_FROM_A", "Descriptive Name"="Search Trigger Edge Copy From A", "Data Type"=4, "Command"="SEAR:TRIG:EDGE:ACOP", "Access"=1, "Range Table"="", "Read Callback"="", "Write Callback"="rsscope_FormatSearchNameEvent_WriteCallback.vi", "Supported Models"="", "Instrument Options"="", "Flags"=0, "Help"="Copies the trigger event configuration from Trigger A for the selected channel source to the search condition settings. Set the selected search name with RSSCOPE_ATTR_SELECTED_SEARCH_NAME.\n\nAvailable Repeated Capabilities:\nNone\n\nRemote-control command(s):\nSEARch:TRIGger:EDGE:ACOPy"}, {"Level"=4, "Class Only"=FALSE, "Identifier"="RSSCOPE_ATTR_SEARCH_TRIGGER_EDGE_COPY_FROM_B", "Descriptive Name"="Search Trigger Edge Copy From B", "Data Type"=4, "Command"="SEAR:TRIG:EDGE:BCOP", "Access"=1, "Range Table"="", "Read Callback"="", "Write Callback"="rsscope_FormatSearchNameEvent_WriteCallback.vi", "Supported Models"="", "Instrument Options"="", "Flags"=0, "Help"="Copies the trigger event configuration from Trigger B for the selected channel source to the search condition settings. Set the selected search name with RSSCOPE_ATTR_SELECTED_SEARCH_NAME.\n\nAvailable Repeated Capabilities:\nNone\n\nRemote-control command(s):\nSEARch:TRIGger:EDGE:BCOPy"}, {"Level"=3, "Class Only"=TRUE, "Identifier"="", "Descriptive Name"="Glitch", "Data Type"=0, "Command"="", "Access"=0, "Range Table"="", "Read Callback"="", "Write Callback"="", "Supported Models"="", "Instrument Options"="", "Flags"=0, "Help"="Configures the conditions for the glitch trigger search.  A glitch trigger occurs when the trigger signal has a pulse with a width that is less than the glitch width.  You specify the glitch width in the Glitch Width parameter.  You specify the polarity of the pulse with the Glitch Polarity
